vi "PID_FPGA.vi"() -> ()   [LabVIEW 2016]
uses:
  <vilib>/rvi/Emulation/niFpgaGetClockAttributes.vi
  <vilib>/rvi/Emulation/niFpgaSctlEmulationGetInTimedLoop.vi
  <vilib>/rvi/Emulation/niFpgaEmulationReportErrorSimple.vi
  <vilib>/rvi/Emulation/niFpgaProcessEmulError.vi
  <vilib>/rvi/eio/common/nirviEmuTemplateMethod_errors.vi
  <vilib>/rvi/Emulation/niFpgaCriticalErrorInLSC.vi
  <vilib>/eio/EIONode/EIONode.xnode
  <vilib>/addons/control/pid/fpga.llb/XNode/niFpgaPID.xnode
panel:
  out "Temperature Alert R":bool
  out "Brake running/ R":bool
  out "Brake locked / Error R":bool
  out "Output AO R":fxp<+/-,17,6>
  in  "Output range 2":T1={"Output high"=10.0, "Output low"=-10.0}
  in  "PID gains 2":T2={"proportional gain (Kc)"=1.0, "integral gain (Kc*Ts/Ti)"=0.05078125, "derivative gain (Kc*Td/Ts)"=0.0}
  out "Input AI R":fxp<+/-,20,5>
  out "Input AI L":fxp<+/-,20,5>
  in  "reset?":bool
  out "Brake running/ L":bool
  out "Brake locked / Error L":bool
  out "Temperature Alert L":bool
  in  "Mod3/Calibration ON Brake L":bool
  in  "Mod3/Unit ON Brake L":bool
  in  "Mod3/Brake Performance ON Brake L":bool
  in  "Mod3/Control Reset Brake L":bool
  in  "Mod3/Control ON Brake L":bool
  in  "setpoint":fxp<+/-,16,5>
  in  "Output range":T1={"Output high"=10.0, "Output low"=-10.0}
  in  "PID gains":T2={"proportional gain (Kc)"=1.0, "integral gain (Kc*Ts/Ti)"=0.05078125, "derivative gain (Kc*Td/Ts)"=0.0}
  in  "Count(mSec)":u32=25
  in  "Alarm ON":bool
  out "Output AO L":fxp<+/-,33,22>
  in  "PID Brake L":bool
  in  "Mod3/System Reset/ON":bool
  in  "STOP":bool
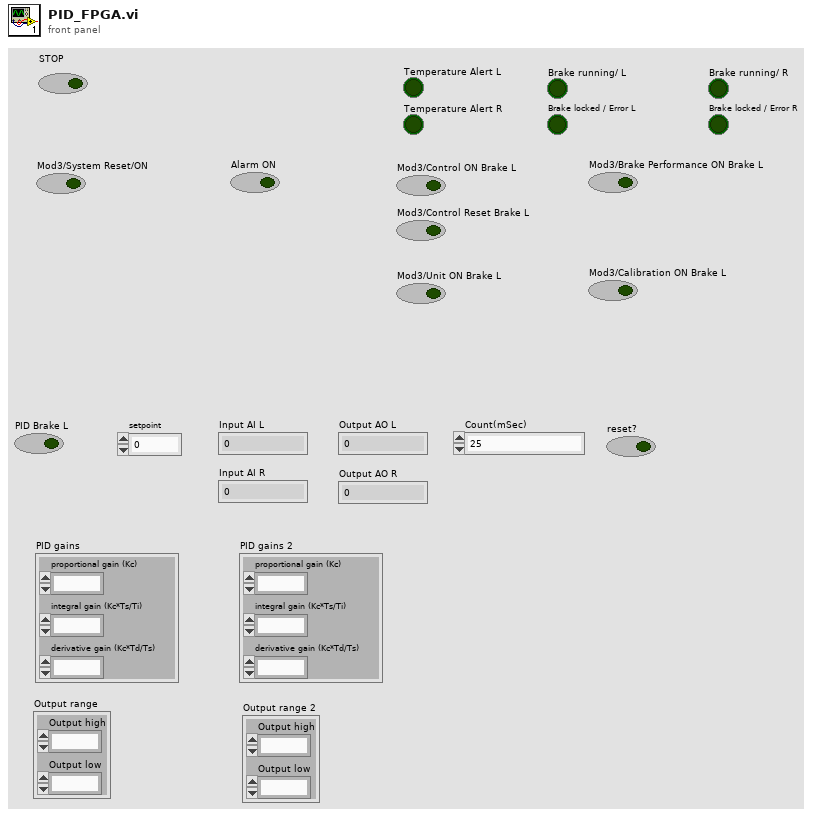
[diagram p1: front panel]
types:
  T1 = cluster{"Output high":fxp<+/-,16,5>, "Output low":fxp<+/-,16,5>}
  T2 = cluster{"proportional gain (Kc)":fxp<+/-,16,8>, "integral gain (Kc*Ts/Ti)":fxp<+/-,16,8>, "derivative gain (Kc*Td/Ts)":fxp<+/-,16,8>}
  T3 = cluster{"proportional gain (Kc)":i16, "integral gain (Kc*Ts/Ti)":i16, "derivative gain (Kc*Td/Ts)":i16}
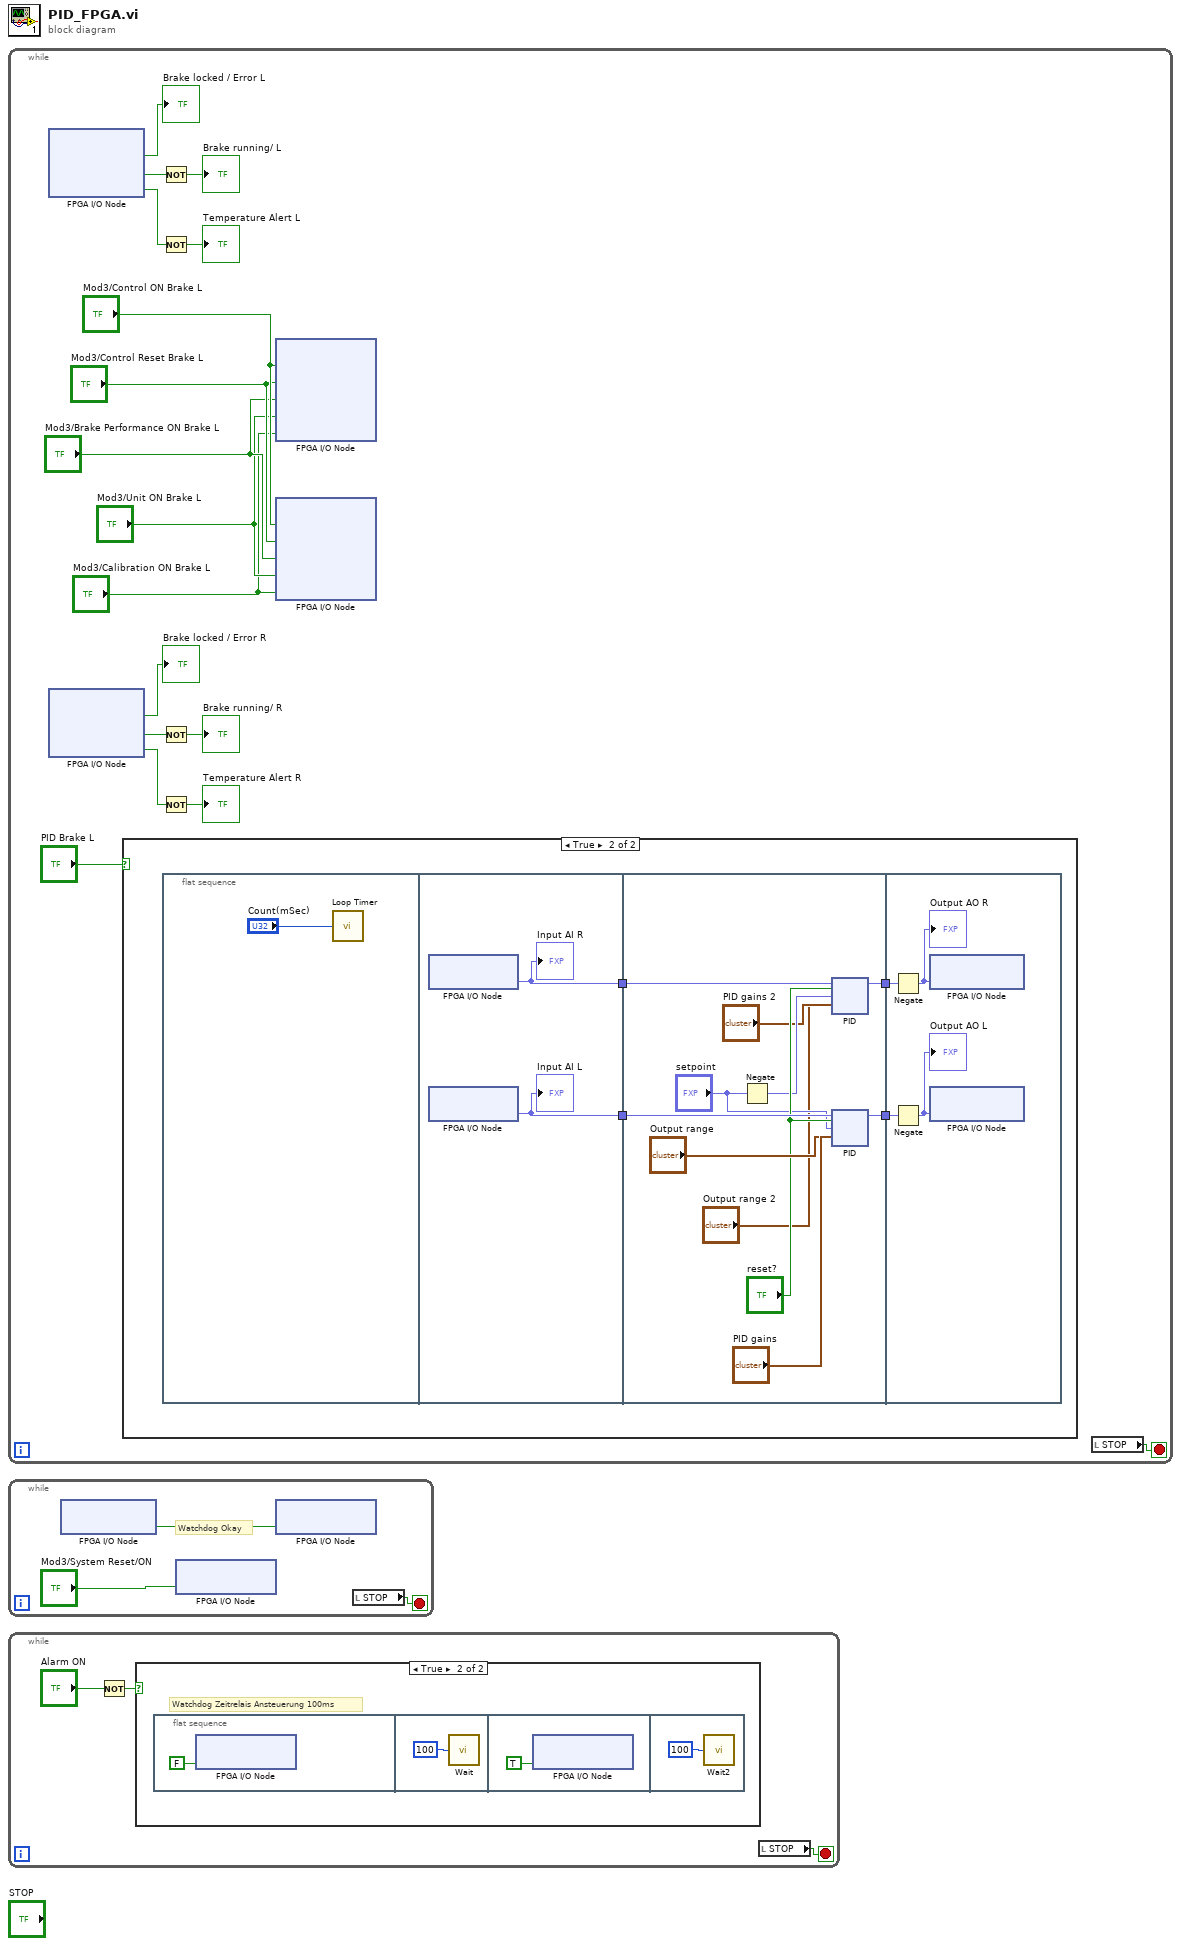
[diagram p0: block diagram]
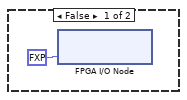
[diagram p3: hidden frame]
diagram:
  n1 = while {
    stop <- w17 stop-if-true
    n2 = xnode "FPGA I/O Node"() -> ("Mod5/DI8"=→"Brake locked / Error L":bool, "Mod5/DI9"=w12:bool, "Mod5/DI10"=w15:bool)  [unwired: 3 in, 3 out]
    n3 = xnode "FPGA I/O Node"() -> ("Mod5/DI24"=→"Brake locked / Error R":bool, "Mod5/DI25"=w9:bool, "Mod5/DI26"=w7:bool)  [unwired: 3 in, 3 out]
    n4 = case shown="True" "PID Brake L" {
      frame False {
        n5 = xnode "FPGA I/O Node"("Mod1/AO2"=fxp<+/-,20,5> 0.0) -> ()  [unwired: 1 in, 1 out]
      }
      frame True {
        n6 = flat-sequence {
          tunnel: [w25] -> w21
          tunnel: [w24] -> w20
          tunnel: [w35] -> w22
          tunnel: w21 -> [w33]
          tunnel: w20 -> [w32]
          tunnel: [w26] -> w19
          tunnel: w22 -> [w96]
          tunnel: w19 -> [w94]
          frame #0 {
            n7 = call "Loop Timer"("Count(mSec)"="Count(mSec)") -> ()  [unwired: 1 out]
          }
          frame #1 {
            n8 = xnode "FPGA I/O Node"() -> ("Mod2/AI1"=w24:fxp<+/-,20,5>)  [unwired: 1 in, 1 out]
            "Input AI R" <- w24
            n9 = xnode "FPGA I/O Node"() -> ("Mod2/AI0"=w25:fxp<+/-,20,5>)  [unwired: 1 in, 1 out]
            "Input AI L" <- w25
          }
          frame #2 {
            n10 = Negate(x="setpoint") -> (-x=w29:fxp<+/-,16,5>)
            n11 = xnode "PID"("process variable"=w32, "reset?"="reset?", "setpoint"=w29, "PID gains"="PID gains 2", "output range"="Output range 2") -> ("output"=w26:fxp<+/-,16,5>)
            n12 = xnode "PID"("process variable"=w33, "reset?"="reset?", "setpoint"="setpoint", "PID gains"="PID gains", "output range"="Output range") -> ("output"=w35:fxp<+/-,16,5>)
          }
          frame #3 {
            n13 = Negate(x=w94) -> (-x=w93:fxp<+/-,17,6>)
            "Output AO R" <- w93
            n14 = Negate(x=w96) -> (-x=w95:fxp<+/-,17,6>)
            "Output AO L" <- w95
            n15 = xnode "FPGA I/O Node"("Mod1/AO1"=w93) -> ()  [unwired: 1 in, 1 out]
            n16 = xnode "FPGA I/O Node"("Mod1/AO0"=w95) -> ()  [unwired: 1 in, 1 out]
          }
        }
      }
    }
    n17 = Not(x=w12) -> (.not. x?=→"Brake running/ L":bool)
    n18 = Not(x=w15) -> (.not. x?=→"Temperature Alert L":bool)
    n19 = Not(x=w9) -> (.not. x?=→"Brake running/ R":bool)
    n20 = Not(x=w7) -> (.not. x?=→"Temperature Alert R":bool)
    n21 = xnode "FPGA I/O Node"("Mod3/DO8"="Mod3/Control ON Brake L", "Mod3/DO9"="Mod3/Control Reset Brake L", "Mod3/DO10"="Mod3/Brake Performance ON Brake L", "Mod3/DO11"="Mod3/Unit ON Brake L", "Mod3/DO12"="Mod3/Calibration ON Brake L") -> ()  [unwired: 5 in, 5 out]
    n22 = xnode "FPGA I/O Node"("Mod3/DO24"="Mod3/Control ON Brake L", "Mod3/DO25"="Mod3/Control Reset Brake L", "Mod3/DO26"="Mod3/Brake Performance ON Brake L", "Mod3/DO27"="Mod3/Unit ON Brake L", "Mod3/DO28"="Mod3/Calibration ON Brake L") -> ()  [unwired: 5 in, 5 out]
    n23 = local read "STOP"() -> (w17:bool)
  }
  n24 = while {
    stop <- w98 stop-if-true
    # "Watchdog Okay"
    n25 = xnode "FPGA I/O Node"() -> ("Mod6/DI16"=w99:bool)  [unwired: 1 in, 1 out]
    n26 = xnode "FPGA I/O Node"("Mod3/DO16"="Mod3/System Reset/ON") -> ()  [unwired: 1 in, 1 out]
    n27 = xnode "FPGA I/O Node"("Mod4/DO17"=w99) -> ()  [unwired: 1 in, 1 out]
    n28 = local read "STOP"() -> (w98:bool)
  }
  n29 = while {
    stop <- w101 stop-if-true
    n30 = Not(x="Alarm ON") -> (.not. x?=w102:bool)
    n31 = case shown="True" w102 {
      frame False {
      }
      frame True {
        # "Watchdog Zeitrelais Ansteuerung 100ms"
        n32 = flat-sequence {
          frame #0 {
            n33 = xnode "FPGA I/O Node"("Mod4/DO16"=FALSE) -> ()  [unwired: 1 in, 1 out]
          }
          frame #1 {
            n34 = call "Wait"("Count(mSec)"=u32 100) -> ()  [unwired: 1 out]
          }
          frame #2 {
            n35 = xnode "FPGA I/O Node"("Mod4/DO16"=TRUE) -> ()  [unwired: 1 in, 1 out]
          }
          frame #3 {
            n36 = call "Wait2"("Count(mSec)"=u32 100) -> ()  [unwired: 1 out]
          }
        }
      }
    }
    n37 = local read "STOP"() -> (w101:bool)
  }
